vi "Gumball State Diagram.vi"   [LabVIEW 2013]
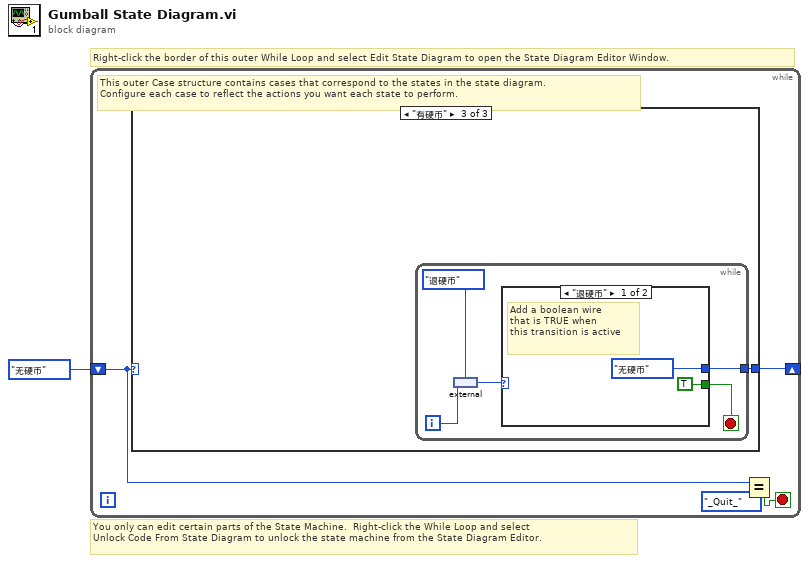
[diagram p0: block diagram]
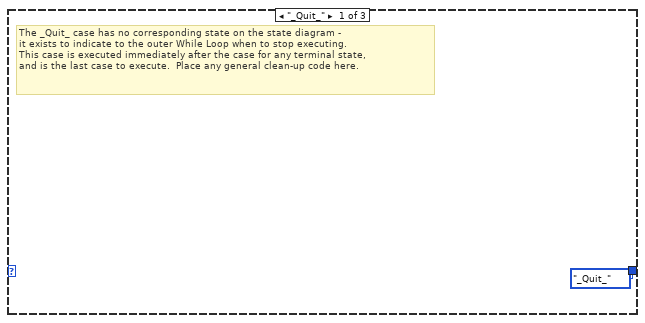
[diagram p2: hidden frame]
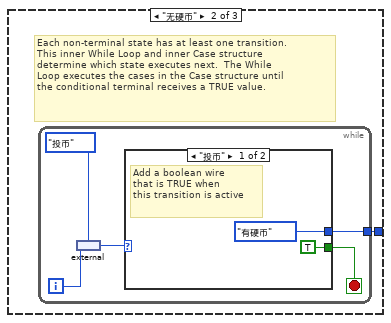
[diagram p3: hidden frame]
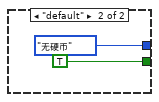
[diagram p4: hidden frame]
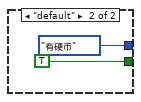
[diagram p5: hidden frame]
diagram:
  # "You only can edit certain parts of the State Machine.  Right-click the While Loop and select \nUnlock Code From State Diagram to unlock the state machine from the State Diagram Editor."
  # "Right-click the border of this outer While Loop and select Edit State Diagram to open the State Diagram Editor Window."
  n1 = while {
    shift-right: [w4] -> _
    shift-left: enum16{"_Quit_", "无硬币", "有硬币"}."无硬币" -> [w5]
    stop <- w3 stop-if-true
    # "This outer Case structure contains cases that correspond to the states in the state diagram.  \nConfigure each case to reflect the actions you want each state to perform."
    n2 = case shown="\"有硬币\"" w5 {
      tunnel: [enum16{"_Quit_", "无硬币", "有硬币"}."_Quit_" w7 w22] -> w4
      frame "_Quit_" {
        # "The _Quit_ case has no corresponding state on the state diagram -\nit exists to indicate to the outer While Loop when to stop executing.\nThis case is executed immediately after the case for any terminal state, \nand is the last case to execute.  Place any general clean-up code here."
      }
      frame "无硬币" {
        # "Each non-terminal state has at least one transition.\nThis inner While Loop and inner Case structure \ndetermine which state executes next.  The While \nLoop executes the cases in the Case structure until \nthe conditional terminal receives a TRUE value."
        n3 = while {
          tunnel: [w9] -> w7
          i -> [w12]
          stop <- w8 stop-if-true
          n4 = external ("Integer to Enum")(enum16{"投币", "default"}."投币", w12) -> (w10:enum16{"投币", "default"})
          n5 = case shown="\"投币\"" w10 {
            tunnel: [enum16{"_Quit_", "无硬币", "有硬币"}."有硬币" enum16{"_Quit_", "无硬币", "有硬币"}."无硬币"] -> w9
            tunnel: [TRUE TRUE] -> w8
            frame "投币" {
              # "Add a boolean wire\nthat is TRUE when\nthis transition is active"
            }
            frame "default" {
            }
          }
        }
      }
      frame "有硬币" {
        n6 = while {
          tunnel: [w24] -> w22
          i -> [w27]
          stop <- w23 stop-if-true
          n7 = external ("Integer to Enum")(enum16{"退硬币", "default"}."退硬币", w27) -> (w25:enum16{"退硬币", "default"})
          n8 = case shown="\"退硬币\"" w25 {
            tunnel: [enum16{"_Quit_", "无硬币", "有硬币"}."无硬币" enum16{"_Quit_", "无硬币", "有硬币"}."有硬币"] -> w24
            tunnel: [TRUE TRUE] -> w23
            frame "退硬币" {
              # "Add a boolean wire\nthat is TRUE when\nthis transition is active"
            }
            frame "default" {
            }
          }
        }
      }
    }
    n9 = Equal?(x=w5, y=enum16{"_Quit_", "无硬币", "有硬币"}."_Quit_") -> (x = y?=w3:bool)
  }
